vi "Extract Object (static).vi"(7 "Copy":bool caption="Copy data instead of extracting", 8 "error in (no error)":errorcluster, 11 "ObjMessage in":refnum<class "MSG.lvclass">) -> (0 "error out":errorcluster, 1 "Object":refnum<class>, 2 "Label":string, 3 "ObjMessage out":refnum<class "MSG.lvclass">)   [LabVIEW 2011, in "Messenging.lvlib" / "MSG.lvclass"]
uses:
  MSG.lvclass
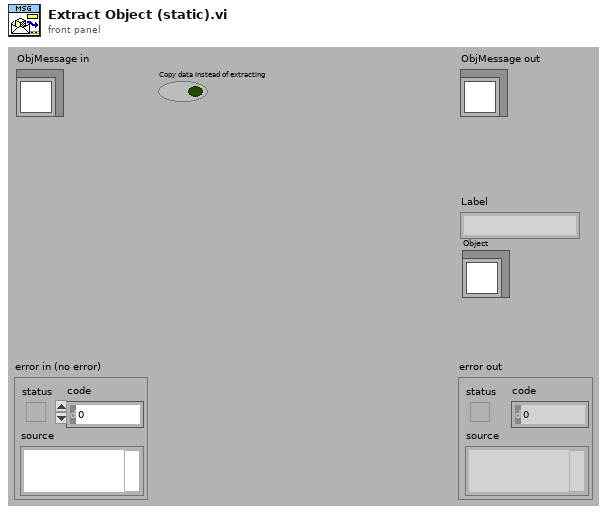
[diagram p1: front panel]
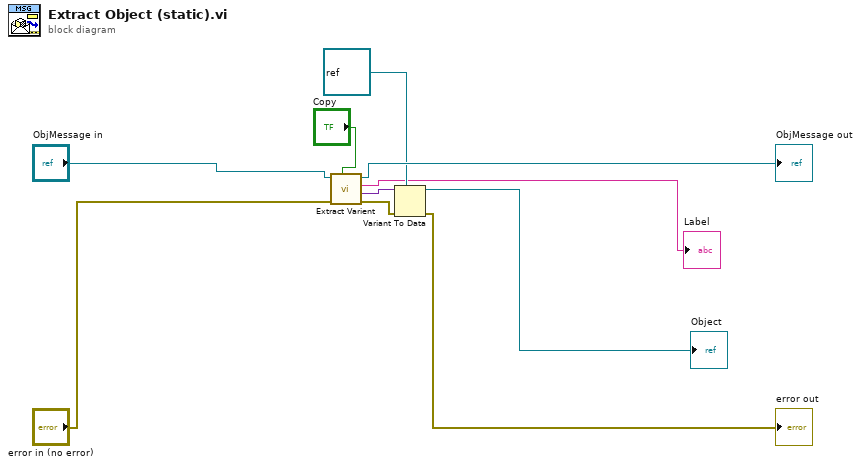
[diagram p0: block diagram]
diagram:
  n1 = call-dynamic "Extract Varient.vi"("Copy"="Copy", "error in (no error)"="error in (no error)", "Message"="ObjMessage in") -> ("error out"=w9:errorcluster, "Varient"=w10:variant, "Label"=→"Label":string, "Message"=→"ObjMessage out":refnum<class "MSG.lvclass">)  [unwired: 5 out]
  n2 = Variant To Data(error in=w9, type=refnum<class> refnum ("Object"), Variant=w10) -> (data=→"Object":refnum<class>, error out=→"error out":errorcluster)
